vi "AOR.vi"(1 "Length":dbl, 2 "Width":dbl) -> (0 "Output":dbl)   [LabVIEW 2017]
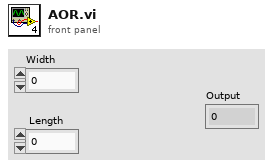
[diagram p1: front panel]
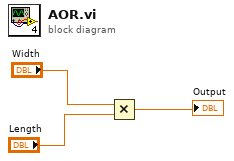
[diagram p0: block diagram]
diagram:
  n1 = Multiply(x="Width", y="Length") -> (x*y=→"Output":dbl)
